vi "emi_SMLoop Control.vi"   [LabVIEW 2011]
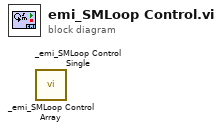
[diagram p0: block diagram]
diagram:
  n1 = call "_emi_SMLoop Control Array.vi"() -> ()  [unwired: 14 in, 2 out]
  n2 = call "_emi_SMLoop Control Single.vi"() -> ()  [unwired: 14 in, 2 out]
